vi "Abort.vi"(8 "error in (no error)":errorcluster, 11 "JKI SMO in":refnum<class "JKI SMO.lvclass">) -> (0 "error out":errorcluster, 3 "JKI SMO out":refnum<class "JKI SMO.lvclass">)   [LabVIEW 2013, in "JKI SMO.lvclass"]
doc: "---------------------------------------------------------------\nJKI State Machine Objects™\nhttp://jki.net/state-machine-objects/\nCopyright (C) 2005-2015, JKI <info@jki.net>\nALL RIGHTS RESERVED"
uses:
  JKI SMO.lvclass
  JKI SMO.lvclass/JKI SMO.ctl
panel:
  # "For instructions on how to use the JKI State Machine Objects, examples and video tutorials, visit:\nhttp://jki.net/state-machine-objects/\n\nJKI State Machine Objects™\nhttp://jki.net/state-machine-objects/\nCopyright (C) 2005-2015, JKI <info@jki.net>\nALL RIGHTS RESERVED"
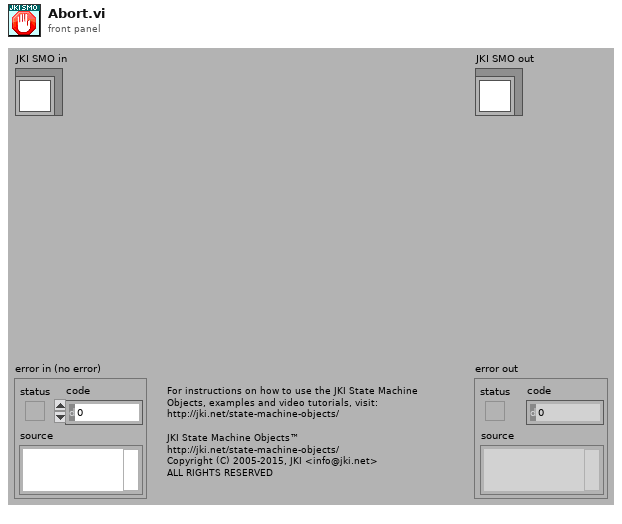
[diagram p1: front panel]
types:
  T1 = typedef "pSubSystem.lvclass/pSubSystem.PrivateData--Cluster.ctl" = cluster{"Processes Clone VI Ref [ ]":refnum<vi>[], "Processes Clone Name [ ]":string[], "Process Sync RendezVous":T2, "Protected Events":T3}
  T2 = typedef "Rendezvous RefNum" = refnum<k1>
  T3 = typedef "pSubSystem.lvclass/pSubSystem.ProtectedEvents--Cluster.ctl" = cluster{"StopProcesses":refnum<user-event>, "AbortProcesses":refnum<user-event>}
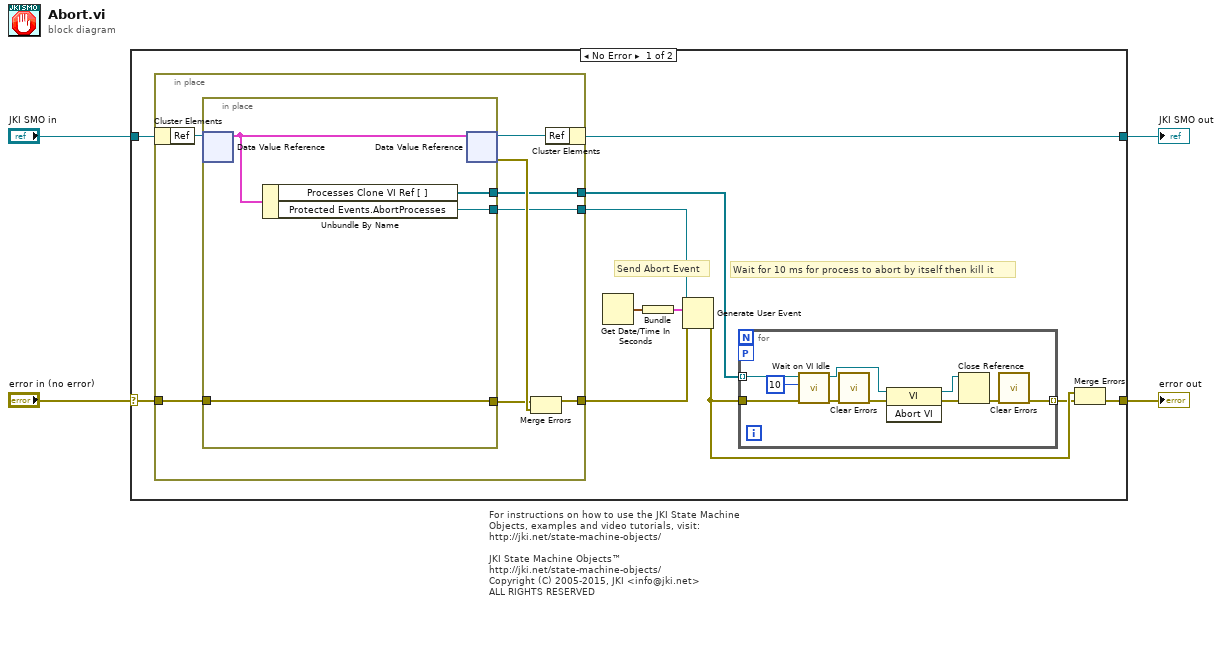
[diagram p0: block diagram]
diagram:
  # "For instructions on how to use the JKI State Machine Objects, examples and video tutorials, visit:\nhttp://jki.net/state-machine-objects/\n\nJKI State Machine Objects™\nhttp://jki.net/state-machine-objects/\nCopyright (C) 2005-2015, JKI <info@jki.net>\nALL RIGHTS RESERVED"
  n1 = case shown="No Error" "error in (no error)" {
    selector: "error in (no error)" -> [w14 w39]
    tunnel: [w6 w39] -> w3
    tunnel: [w13 w38] -> w1
    tunnel: "JKI SMO in" -> [w15 w38]
    frame No Error {
      # "Wait for 10 ms for process to abort by itself then kill it"
      # "Send Abort Event"
      n2 = in-place {
        in-place-border: w14 -> [w32]
        in-place-border: [w29] -> w9
        in-place-border: [w27] -> w10
        in-place-border: [w26] -> w8
        n3 = in-place-cluster #1(w15) -> ("Ref"=w33:refnum<data-value>)
        n4 = in-place {
          in-place-border: w32 -> [w36]
          in-place-border: [w36] -> w30
          in-place-border: [w35] -> w27
          in-place-border: [w34] -> w26
          n5 = in-place-dvr #2(w33) -> (w37:T1)  [unwired: 1 out]
          n6 = Unbundle By Name(w37) -> ("Processes Clone VI Ref [ ]"=w34:refnum<vi>[], "Protected Events.AbortProcesses"=w35:refnum<user-event>)
          n7 = in-place-dvr #2(w37) -> (w28:refnum<data-value>, w31:errorcluster)
        }
        n8 = Merge Errors(w30, w31) -> (w29:errorcluster)
        n9 = in-place-cluster #1("Ref"=w28) -> (w13:refnum<class "JKI SMO.lvclass">)
      }
      n10 = Get Date/Time In Seconds() -> (seconds since 1Jan1904=w11:timestamp)
      n11 = Bundle("seconds since 1Jan1904"=w11) -> (w12:cluster{"seconds since 1Jan1904":timestamp})  [unwired: 1 in]
      n12 = Generate User Event(user event=w10, event data cluster=w12, error in=w9) -> (error out=w7:errorcluster)  [unwired: 1 in, 1 out]
      n13 = for {
        tunnel: w7 -> [w25]
        tunnel: w8 -> [w24] mode=indexing
        workers-P: _ -> [_]
        tunnel: [w19] -> w5 mode=indexing
        n14 = call "Wait on VI Idle.vi"("error in (no error)"=w25, "ms Timout (100ms)"=u32 10, "VI to Wait on"=w24) -> ("error out"=w21:errorcluster, "VI to Wait on dup"=w22:refnum<vi>)  [unwired: 6 in, 1 out]
        n15 = call <vilib>:"Clear Errors.vi"("error in (no error)"=w21) -> ("error out"=w20:errorcluster)  [unwired: 6 in]
        n16 = invoke class="VI" method="Abort VI"(reference=w22, error in=w20) -> (reference out=w16:refnum<vi>, error out=w18:errorcluster)  [unwired: 1 in, 1 out]
        n17 = Close Reference(reference=w16, error in (no error)=w18) -> (error out=w17:errorcluster)
        n18 = call <vilib>:"Clear Errors.vi"("error in (no error)"=w17) -> ("error out"=w19:errorcluster)  [unwired: 6 in]
      }
      n19 = Merge Errors(w7, w5) -> (w6:errorcluster)
    }
    frame Error {
    }
  }
  "error out" <- w3
  "JKI SMO out" <- w1
